vi "draw waveform.vi"() -> ()   [LabVIEW 2009]
uses:
  <vilib>/sound/lvsound.llb/Sound Format.ctl
  <vilib>/gmath/NI_Gmath.lvlib
panel:
  in  "i/s":sgl
  in  "points":i32(slide) scale=3.0..43.0
  in  "Array":dbl[](array[slide]) min=-1.0 max=1.0 scale=-1.0..1.0
  in  "cycles/s":sgl
  in  "stop":bool
  in  "player controls":cluster{"play/pause":bool, "volume":dbl}={"play/pause"=FALSE, "volume"=1.0} {"volume" scale=0.0037..1.0}
  out "Waveform graph":i16[](graph)
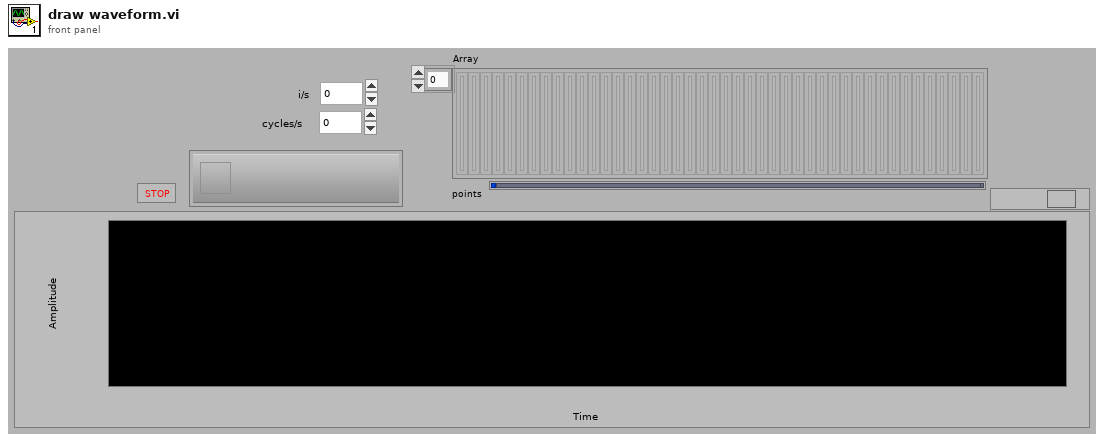
[diagram p1: front panel]
types:
  T1 = typedef "Sound Format.ctl" = cluster{"sound quality":enum16{"mono", "stereo"}, "rate":enum16{"11025", "22050", "44100", "8000"}, "bits per sample":enum16{"8 bit", "16 bit"}}
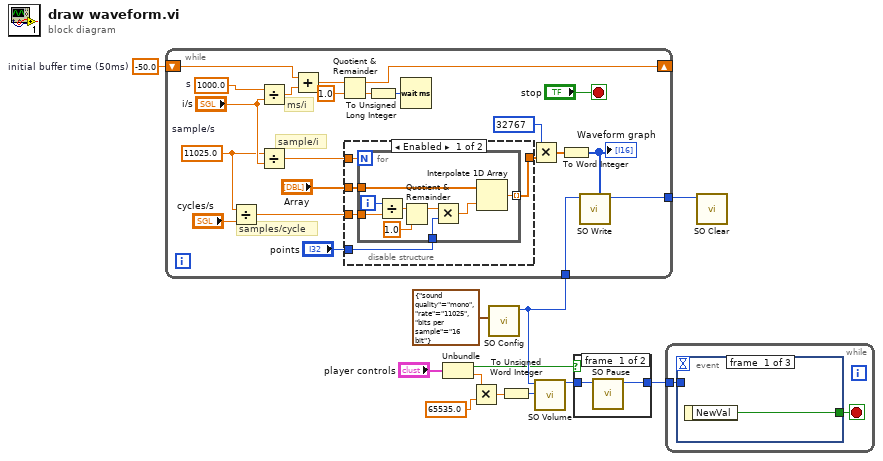
[diagram p0: block diagram]
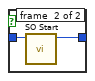
[diagram p2: hidden frame]
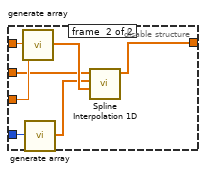
[diagram p3: hidden frame]
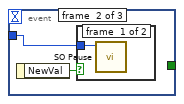
[diagram p4: hidden frame]
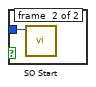
[diagram p5: hidden frame]
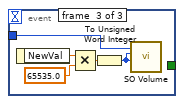
[diagram p6: hidden frame]
diagram:
  w2 = sgl -50.0  # initial buffer time (50ms)
  n1 = Unbundle("player controls") -> ("play/pause"=w5:bool, "volume"=w4:dbl)
  n2 = Multiply(x=w4, y=65535.0 ("left channel")) -> (x*y=w7:dbl)
  n3 = call <vilib>:"SO Config.vi"("sound format"=T1 {"sound quality"=enum."mono", "rate"=enum."11025", "bits per sample"=enum."16 bit"}) -> ("task ID out"=w10:u32)  [unwired: 9 in, 1 out]
  n4 = while {
    tunnel: w10 -> [w33]
    shift-right: [w17] -> _
    shift-left: w2 -> [w15]
    tunnel: [w13] -> w1
    stop <- "stop" stop-if-true
    w27 = sgl 1000.0  # s
    w23 = sgl 11025.0  # sample/s
    # "samples/cycle"
    # "sample/i"
    # "ms/i"
    n5 = Divide(x=w23, y="cycles/s") -> (x/y=w22:sgl)
    n6 = Divide(x=w27, y="i/s") -> (x/y=w16:sgl)
    n7 = Divide(x=w23, y="i/s") -> (x/y=w25:sgl)
    n8 = Add(x=w15, y=w16) -> (x+y=w14:sgl)
    n9 = Quotient & Remainder(x=w14, y=sgl 1.0) -> (x-y*floor(x/y)=w17:sgl, floor(x/y)=w18:sgl)
    n10 = disable-structure shown="Enabled" {
      disable-tunnel: "Array" -> [w39 w50]
      disable-tunnel: [w38 w49] -> w29
      disable-tunnel: w25 -> [w37 w55]
      disable-tunnel: w22 -> [w36 w54]
      disable-tunnel: "points" -> [w35 w53]
      frame #0 {
        n11 = for {
          N: w37 -> [_]
          tunnel: w39 -> [w48]
          tunnel: [w47] -> w38 mode=indexing
          tunnel: w36 -> [w45]
          tunnel: w35 -> [w40]
          i -> [w46]
          n12 = Divide(x=w46, y=w45) -> (x/y=w44:sgl)
          n13 = Quotient & Remainder(x=w44, y=sgl 1.0) -> (x-y*floor(x/y)=w42:sgl)  [unwired: 1 out]
          n14 = Multiply(x=w42, y=w40) -> (x*y=w41:sgl)
          n15 = Interpolate 1D Array(1:w41, 2:w48) -> (0:w47:dbl)
        }
      }
      frame #1 {
        n16 = call "generate array.vi"("size"=w55, "increment"=w54) -> ("Array"=w52:dbl[])  [unwired: 25 in]
        n17 = call "generate array.vi"("size"=w53) -> ("Array"=w51:dbl[])  [unwired: 26 in]
        n18 = call <vilib>:"Spline Interpolation 1D.vi"("xi"=w52, "X"=w51, "Y"=w50) -> ("yi"=w49:dbl[])  [unwired: 6 in, 2 out]
      }
    }
    n19 = To Unsigned Long Integer(number=w18) -> (unsigned 32bit integer=w21:u32)
    n20 = Wait (ms)(milliseconds to wait=w21) -> ()  [unwired: 1 out]
    n21 = Multiply(x=i16 32767, y=w29) -> (x*y=w31:dbl[])
    n22 = To Word Integer(number=w31) -> (16bit integer=w28:i16[])
    "Waveform graph" <- w28
    n23 = call <vilib>:"SO Write.vi"("mono 16-bit"=w28, "task ID in"=w33) -> ("task ID out"=w13:u32)  [unwired: 8 in, 1 out]
  }
  n24 = To Unsigned Word Integer(number=w7) -> (unsigned 16bit integer=w8:u16)
  n25 = call <vilib>:"SO Volume.vi"("left channel"=w8, "task ID in"=w10) -> ("task ID out"=w11:u32)  [unwired: 8 in, 1 out]
  n26 = case shown="True" w5 {
    tunnel: w11 -> [w57 w59]
    tunnel: [w56 w58] -> w3
    frame #0 {
      n27 = call <vilib>:"SO Pause.vi"("task ID in"=w57) -> ("task ID out"=w56:u32)  [unwired: 9 in, 1 out]
    }
    frame #1 {
      n28 = call <vilib>:"SO Start.vi"("task ID in"=w59) -> ("task ID out"=w58:u32)  [unwired: 9 in, 1 out]
    }
  }
  n29 = while {
    tunnel: w3 -> [w60]
    stop <- w61 stop-if-true
    n30 = event shown="[1] \"player controls.play/pause\": Value Change" {
      selector: _ -> [_ _ _]
      dyn-events: _ -> [_ _ _]
      timeout: _ -> [_ _ _]
      tunnel: [w62 _ _] -> w61
      tunnel: w60 -> [_ w63 w67]
      event #0 {
        n31 = event-data() -> ("NewVal"=w62:bool)  [unwired: 1 in]
      }
      event #1 {
        n32 = event-data() -> ("NewVal"=w64:bool)  [unwired: 1 in]
        n33 = case shown="True" w64 {
          tunnel: w63 -> [w65 w66]
          frame #0 {
            n34 = call <vilib>:"SO Pause.vi"("task ID in"=w65) -> ()  [unwired: 9 in, 2 out]
          }
          frame #1 {
            n35 = call <vilib>:"SO Start.vi"("task ID in"=w66) -> ()  [unwired: 9 in, 2 out]
          }
        }
      }
      event #2 {
        n36 = event-data() -> ("NewVal"=w71:dbl)  [unwired: 1 in]
        n37 = Multiply(x=w71, y=65535.0 ("left channel")) -> (x*y=w69:dbl)
        n38 = To Unsigned Word Integer(number=w69) -> (unsigned 16bit integer=w70:u16)
        n39 = call <vilib>:"SO Volume.vi"("right channel"=w70, "left channel"=w70, "task ID in"=w67) -> ()  [unwired: 7 in, 2 out]
      }
    }
  }
  n40 = call <vilib>:"SO Clear.vi"("task ID in"=w1) -> ()  [unwired: 10 in, 1 out]
